vi "PH_Countdown-Counter.constructor.vi"(0 "name":string, 2 "data in":string, 5 "error in(no error)":errorcluster) -> (14 "i ref out":refnum<vi>, 16 "data out":string, 19 "error out":errorcluster)   [LabVIEW 2014, in "PH_Countdown-Counter.lvlib"]
doc: "The Sequencer controlles the PHELIX shot procedure.\n\nThis class is part of the PHELIX user layer.\n\nauthor: Stefan Götte, GSI\n\nLicense Agreement for this software:\n\nCopyright (C)\nGesellschaft für Schwerionenforschung, GSI\nPlanckstr. 1\n64291 Darmstadt\nGermany\n\nContact: D.Beck@gsi.de \n\nThis program is free software; you can redistribute it and/or modify it under the terms of the \nGNU General Public License as published by the Free Software Foundation; either version 2 of \nthe license, or (at your option) any later version.\n\nThis program is distributed in the hope that it will be useful, but WITHOUT ANY WARRANTY; \nwithout even the implied warranty of MERCHANTABILITY or FITNESS FOR A PARTICULAR PURPOSE. See the GNU General License for more details (http://www.gnu.org).\n\nGesellschaft für Schwerionenforschung, GSI\nPlanckstr. 1, 64291 Darmstadt, Germany\nFor all questions and ideas contact: M.Richter@gsi.de, H.Brand@gsi.de or D.Beck@gsi.de.\nLast update: 16-JUN-2004"
uses:
  PH_Countdown-Counter.lvlib
  PH_Countdown-Counter.i attribute.ctl
  PH_Basics/PH_PP_Common/PH_PP_Common.PUs.ctl
  PH_Basics/PH_PowerUnit_BaseClass/PH_PowerUnit_BaseClass.PP PU Tags.ctl
  PH_Basics/PH_PP_Common/PH_PP_Common.Trigger Tags.ctl
  PH_Basics/PH_Common/PH_Common.lvlib
  CS_Core/CSObj/CSObj.lvlib
  PH_Basics/PH_PowerUnit_BaseClass/PH_PowerUnit_BaseClass.lvlib
  PH_Basics/PH_PP_Common/PH_PP_Common.lvlib
  PH_Basics/PH_Class/PH_Class.lvlib
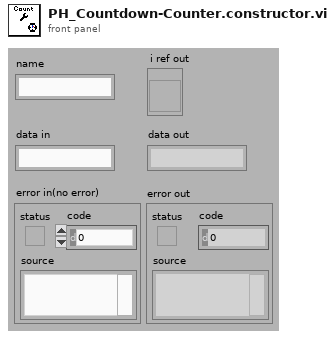
[diagram p1: front panel]
types:
  T1 = typedef "PH_Countdown-Counter.lvlib/PH_Countdown-Counter.i attribute.ctl" = cluster{"Machine Time":cluster{"Tag":string, "Wating Time [s]":dbl, "not linked?":bool}[], "Last Shot":cluster{"Tag":string, "Shot Time [s]":timestamp, "not linked?":bool}[], "Time since last Shot?":bool, "Calculation":cluster{"Time between Shots [s]":dbl, "Ref Remaining Time":refnum<vi>, "Service ID":i32, "over?":bool, "Ref Time between Shots":refnum<vi>, "Ref Set Mode":refnum<vi>}, "Sound?":bool, "Reminder":cluster{"# 1":cluster{"Pretime [s]":dbl, "Aktive?":bool, "Over?":bool}, "# 2":cluster{"Pretime [s]":dbl, "Aktive?":bool, "Over?":bool}}, "MainAmp only":cluster{"State":bool, "GUI Ref":refnum<vi>}}
  T2 = enum16{"SetAttribute", "GetAttribute", "CreateAttribute", "DestroyAttribute", "DestroyAllAtributes"}
  T3 = typedef "PH_PP_Common.lvlib/PH_PP_Common.Trigger Tags.ctl" = enum16{"triggered", "fired", "Status", "Last Shot"}
  T4 = typedef "PH_PowerUnit_BaseClass.lvlib/PH_PowerUnit_BaseClass.PP PU Tags.ctl" = enum16{"Waiting-Time", "PU-in-Use"}
  T5 = cluster{"Tag":string, "Wating Time [s]":dbl, "not linked?":bool}
  T6 = cluster{"Tag":string, "Shot Time [s]":timestamp, "not linked?":bool}
  T7 = typedef "PH_PP_Common.lvlib/PH_PP_Common.PUs.ctl" = enum16{"no Info", "PA-19mm-1", "PA-19mm-2", "PA-45mm-PILC", "PA-45mm-MAIN", "MA-PU-1", "MA-PU-2", "MA-PU-3", "MA-PU-4", "MA-PU-5", "MA-PU-6", "MA-FR", "MA-PILC", "PA-45mm-DP"}
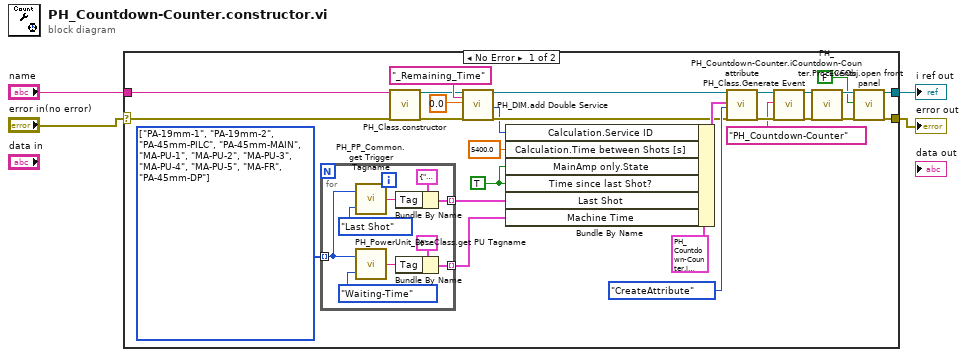
[diagram p0: block diagram]
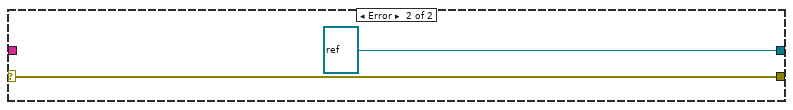
[diagram p2: hidden frame]
diagram:
  n1 = case shown="No Error" "error in(no error)" {
    selector: "error in(no error)" -> [w29 w42]
    tunnel: "name" -> [w30 _]
    tunnel: [w23 w42] -> w3
    tunnel: [w24 refnum<vi> refnum ("i ref out")] -> w2
    frame No Error {
      w11 = T7[] [enum."PA-19mm-1", enum."PA-19mm-2", enum."PA-45mm-PILC", enum."PA-45mm-MAIN", enum."MA-PU-1", enum."MA-PU-2", enum."MA-PU-3", enum."MA-PU-4", enum."MA-PU-5", enum."MA-FR", enum."PA-45mm-DP"] items=["no Info", "PA-19mm-1", "PA-19mm-2", "PA-45mm-PILC", "PA-45mm-MAIN", "MA-PU-1", "MA-PU-2", "MA-PU-3", "MA-PU-4", "MA-PU-5", "MA-PU-6", "MA-FR", "MA-PILC", "PA-45mm-DP"]
      w19 = TRUE ("MainAmp only.State")
      n2 = for {
        tunnel: [w38] -> w13 mode=indexing
        tunnel: [w37] -> w12 mode=indexing
        tunnel: w11 -> [w32] mode=indexing
        n3 = call "PH_PP_Common.get Trigger Tagname.vi"("Trigger Tag"=PH_PP_Common.Trigger_Tags."Last Shot", "PU"=w32) -> ("Trigger Tagname"=w34:string)
        n4 = call "PH_PowerUnit_BaseClass.get PU Tagname.vi"("PU Tag"=PH_PowerUnit_BaseClass.PP_PU_Tags."Waiting-Time", "PU"=w32) -> ("PU Tagname"=w36:string)
        n5 = Bundle By Name(cluster=T6 {"Tag"="", "Shot Time [s]"=timestamp(0 s since 1904-01-01), "not linked?"=FALSE} ("PU"), "Tag"=w34) -> (w38:T6)
        n6 = Bundle By Name(cluster=T5 {"Tag"="", "Wating Time [s]"=0.0, "not linked?"=FALSE} ("PU"), "Tag"=w36) -> (w37:T5)
      }
      n7 = call "PH_Class.constructor.vi"("name"=w30, "error in"=w29) -> ("i ref out"=w16:refnum<vi>, "error out"=w17:errorcluster)  [unwired: 15 in, 1 out]
      n8 = call "PH_DIM.add Double Service.vi"("i ref in"=w16, "Service Name"="_Remaining_Time" ("string"), "Double Value"=0.0, "error in (no error)"=w17) -> ("i ref out"=w15:refnum<vi>, "Service ID"=w10:i32, "error out"=w14:errorcluster)  [unwired: 13 in]
      n9 = Bundle By Name(cluster=T1 {"Machine Time"=[], "Last Shot"=[], "Time since last Shot?"=FALSE, "Calculation"={"Time between Shots [s]"=5400.0, "Ref Remaining Time"=refnum, "Service ID"=-1, "over?"=FALSE, "Ref Time between Shots"=refnum, "Ref Set Mode"=refnum}, "Sound?"=FALSE, "Reminder"={"# 1"={"Pretime [s]"=0.0, "Aktive?"=FALSE, "Over?"=FALSE}, "# 2"={"Pretime [s]"=0.0, "Aktive?"=FALSE, "Over?"=FALSE}}, "MainAmp only"={"State"=TRUE, "GUI Ref"=refnum}} ("i attribute"), "Calculation.Service ID"=w10, "Calculation.Time between Shots [s]"=5400.0, "MainAmp only.State"=w19, "Time since last Shot?"=w19, "Last Shot"=w13, "Machine Time"=w12) -> (w18:T1)
      n10 = call "PH_Countdown-Counter.i attribute.vi"("VI Refnum"=w15, "CLASS.i attribute"=w18, "Action"=T2."CreateAttribute", "error in (no error)"=w14) -> ("VI Refnum out"=w7:refnum<vi>, "error out"=w6:errorcluster)  [unwired: 13 in, 1 out]
      n11 = call "PH_Class.Generate Event.vi"("i ref in"=w7, "Class"="PH_Countdown-Counter", "error in (no error)"=w6) -> ("i ref out"=w9:refnum<vi>, "error out"=w8:errorcluster)  [unwired: 15 in]
      n12 = call "PH_Countdown-Counter.ProcEvents.vi"("i ref in"=w9, "error in (no error)"=w8) -> ("i ref out"=w25:refnum<vi>, "error out"=w26:errorcluster)  [unwired: 16 in]
      n13 = call "CSObj.open front panel.vi"("i ref in"=w25, "frontPanelOpen"=FALSE, "error in (no error)"=w26) -> ("i ref out"=w24:refnum<vi>, "error out"=w23:errorcluster)  [unwired: 15 in]
    }
    frame Error {
    }
  }
  "i ref out" <- w2
  "error out" <- w3
